vi "Action.vi"(8 "error in (no error)":errorcluster, 10 "OOQMH in":refnum<class "OOQMH.lvclass">, 11 "Set Output Range in":refnum<class "Set Output Range.lvclass">) -> (0 "error out":errorcluster, 2 "OOQMH out":refnum<class "OOQMH.lvclass">, 3 "Set Output Range out":refnum<class "Set Output Range.lvclass">)   [LabVIEW 2024, in "PID Loop.lvlib" / "Set Output Range.lvclass"]
uses:
  Set Output Range.lvclass
  OOQMH/OOQMH/OOQMH.lvclass
  PID Loop/PID Loop.lvclass
  C:/Users/uspoaotto/OneDrive - Oregon Tool/Desktop/working copies/helperLoop/src/OOQMH/OOQMH/OOQMH.lvclass
  Set Output Range.lvclass/Set Output Range.ctl
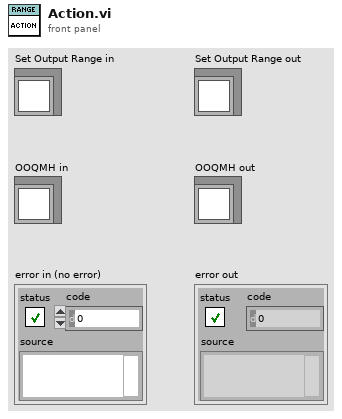
[diagram p1: front panel]
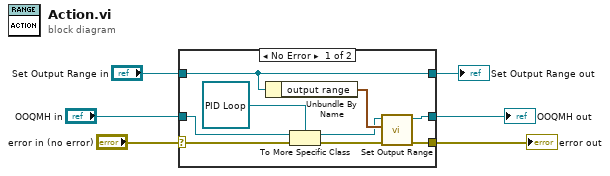
[diagram p0: block diagram]
diagram:
  n1 = case shown="No Error" "error in (no error)" {
    selector: "error in (no error)" -> [w8 w17]
    tunnel: "OOQMH in" -> [w14 w18]
    tunnel: [w11 w18] -> w5
    tunnel: [w10 w17] -> w4
    tunnel: "Set Output Range in" -> [w7 w16]
    tunnel: [w7 w16] -> w1
    frame No Error {
      n2 = Unbundle By Name(w7) -> ("output range"=w15:cluster{"output high":dbl, "output low":dbl})
      n3 = To More Specific Class(target class=refnum<class "PID Loop.lvclass"> refnum ("PID Loop in"), reference=w14, error in=w8) -> (specific class reference=w13:refnum<class "PID Loop.lvclass">, error out=w12:errorcluster)
      n4 = call-dynamic "Set Output Range.vi"("error in (no error)"=w12, "output range"=w15, "PID Loop in"=w13) -> ("error out"=w10:errorcluster, "PID Loop out"=w11:refnum<class "PID Loop.lvclass">)  [unwired: 7 in]
    }
    frame Error {
    }
  }
  "error out" <- w4
  "Set Output Range out" <- w1
  "OOQMH out" <- w5
